vi "Get_Each_channel_reference_samplingdata.vi"(0 "SPU":refnum<k24>, 1 "STSProcess.PDLSTS":refnum<k24>, 2 "Refdata_struct":refnum<k24>[](array[refnum]), 3 "SOP":i32, 5 "Ref_monitordata_struct":refnum<k24>[](array[refnum]), 7 "MPM":refnum<k24>[](array[refnum]), 9 "ChannelNumber":i32, 11 "错误输入（无错误）":errorcluster, 12 "SweepCount":i32, 13 "SlotNumber":i32, 14 "MPMNumber":i32) -> (6 "PDLSTS out":refnum<k24>, 15 "error out":errorcluster)   [LabVIEW 2017]
doc: "Get logging reference data & add in"
uses:
  D:/test/PDLSTS/LV_PDL_Sample/DLL/STSProcess.dll
  DLL/STSProcess.dll
  D:/test/PDLSTS/LV_PDL_Sample/DLL/InstrumentDLL.dll
  DLL/InstrumentDLL.dll
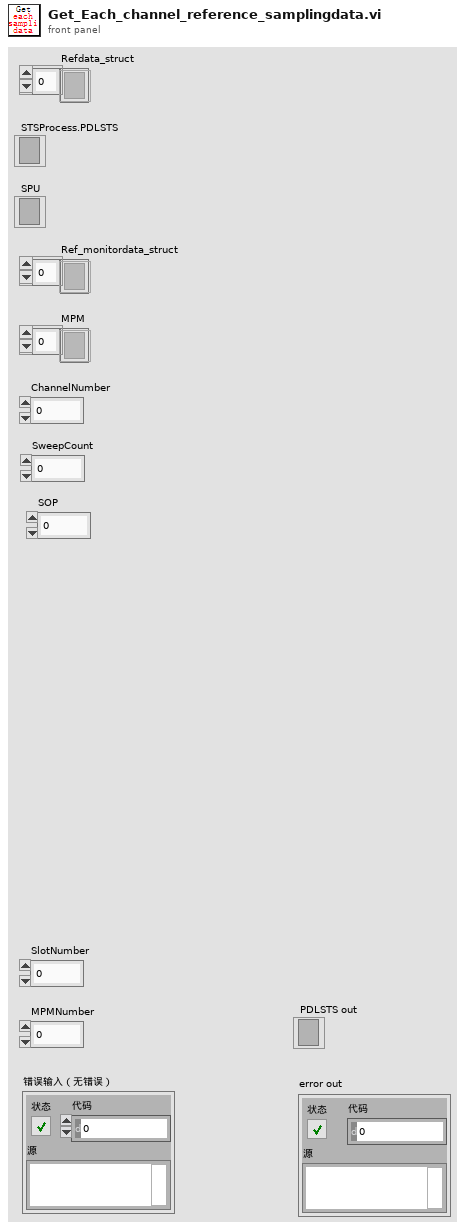
[diagram p1: front panel]
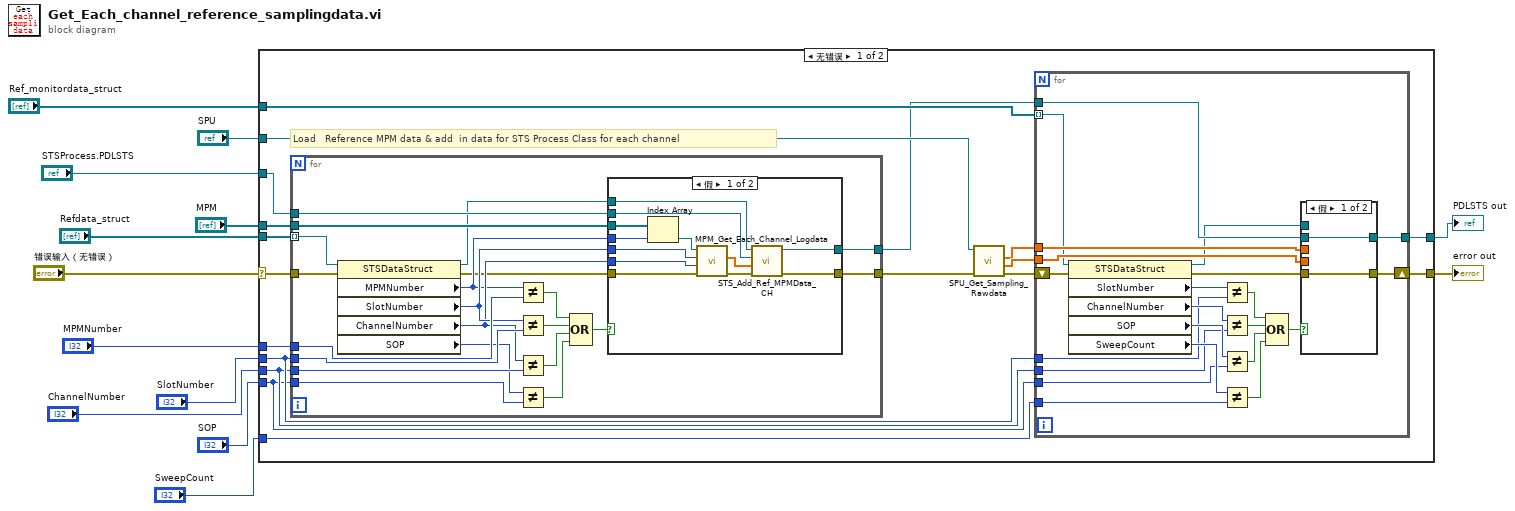
[diagram p0: block diagram]
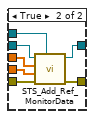
[diagram p2: hidden frame]
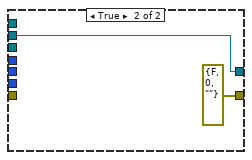
[diagram p3: hidden frame]
diagram:
  n1 = case shown="无错误" "错误输入（无错误）" {
    selector: "错误输入（无错误）" -> [w21 w99]
    tunnel: "STSProcess.PDLSTS" -> [w19 w98]
    tunnel: "Ref_monitordata_struct" -> [w28 _]
    tunnel: "SPU" -> [w27 _]
    tunnel: "MPM" -> [w25 _]
    tunnel: "ChannelNumber" -> [w16 _]
    tunnel: "SlotNumber" -> [w17 _]
    tunnel: "MPMNumber" -> [w24 _]
    tunnel: "Refdata_struct" -> [w23 _]
    tunnel: [w22 w99] -> w5
    tunnel: [w20 w98] -> w3
    tunnel: "SOP" -> [w15 _]
    tunnel: "SweepCount" -> [w14 _]
    frame No Error {
      # "Load　Reference MPM data & add  in data for STS Process Class for each channel"
      n2 = for {
        tunnel: w23 -> [w71] mode=indexing
        tunnel: w24 -> [w83]
        tunnel: w17 -> [w82]
        tunnel: w16 -> [w81]
        tunnel: w25 -> [w74]
        tunnel: w19 -> [w72]
        tunnel: [w70] -> w26
        tunnel: w21 -> [w68]
        tunnel: [w66] -> w18
        tunnel: w15 -> [w64]
        n3 = property on="属性节点" class="STSDataStruct"(reference=w71, error in=w68) -> (reference out=w67:refnum<k24>, error out=w69:errorcluster, "MPMNumber"=w73:i32, "SlotNumber"=w76:i32, "ChannelNumber"=w75:i32, "SOP"=w65:i32)
        n4 = Not Equal?(x=w73, y=w83) -> (x != y?=w80:bool)
        n5 = Not Equal?(x=w76, y=w82) -> (x != y?=w79:bool)
        n6 = Not Equal?(x=w75, y=w81) -> (x != y?=w78:bool)
        n7 = Not Equal?(x=w65, y=w64) -> (x != y?=w63:bool)
        n8 = Compound Arithmetic op=OR ("复合运算")(w80, w79, w78, w63) -> (w77:bool)
        n9 = case shown="假" w77 {
          tunnel: w76 -> [w95 _]
          tunnel: w75 -> [w94 _]
          tunnel: w74 -> [w93 _]
          tunnel: w73 -> [w91 _]
          tunnel: w72 -> [w90 w96]
          tunnel: w67 -> [w89 _]
          tunnel: [w86 errorcluster {"status"=FALSE, "code"=0, "source"=""} ("错误输出")] -> w70
          tunnel: w69 -> [w85 _]
          tunnel: [w84 w96] -> w66
          frame False {
            n10 = Index Array(array=w93, index=w91) -> (element=w92:refnum<k24>)
            n11 = call "MPM_Get_Each_Channel_Logdata.vi"("error in (no error)"=w85, "channelNumber"=w94, "moduleNumber"=w95, ".NET Reference in"=w92) -> ("error out"=w87:errorcluster, "data out"=w88:sgl[])  [unwired: 5 in, 1 out]
            n12 = call "STS_Add_Ref_MPMData_CH.vi"("错误输入（无错误）"=w87, "data"=w88, "STSProcess.PDSTS"=w90, "Setting"=w89) -> ("错误输出"=w86:errorcluster, "PDLSTS"=w84:refnum<k24>)  [unwired: 6 in]
          }
          frame True {
          }
        }
      }
      n13 = call "SPU_Get_Sampling_Rawdata.vi"("错误输入（无错误）"=w26, "SPU"=w27) -> ("error out"=w29:errorcluster, "monitor"=w31:sgl[], "trigger"=w30:sgl[])  [unwired: 5 in, 1 out]
      n14 = for {
        tunnel: w28 -> [w48] mode=indexing
        tunnel: w18 -> [w53]
        tunnel: w30 -> [w52]
        tunnel: w31 -> [w51]
        shift-right: [w50] -> w22
        shift-left: w29 -> [w46]
        tunnel: [w49] -> w20
        tunnel: w17 -> [w35]
        tunnel: w16 -> [w34]
        tunnel: w15 -> [w33]
        tunnel: w14 -> [w32]
        n15 = property class="STSDataStruct"(reference=w48, error in=w46) -> (reference out=w47:refnum<k24>, error out=w45:errorcluster, "SlotNumber"=w39:i32, "ChannelNumber"=w38:i32, "SOP"=w37:i32, "SweepCount"=w36:i32)
        n16 = Not Equal?(x=w39, y=w35) -> (x != y?=w44:bool)
        n17 = Not Equal?(x=w38, y=w34) -> (x != y?=w43:bool)
        n18 = Not Equal?(x=w37, y=w33) -> (x != y?=w42:bool)
        n19 = Not Equal?(x=w36, y=w32) -> (x != y?=w41:bool)
        n20 = Compound Arithmetic op=OR ("复合运算")(w44, w43, w42, w41) -> (w40:bool)
        n21 = case shown="假" w40 {
          tunnel: w53 -> [w55 w62]
          tunnel: w47 -> [_ w61]
          tunnel: w52 -> [_ w60]
          tunnel: w51 -> [_ w59]
          tunnel: w45 -> [w54 w58]
          tunnel: [w54 w57] -> w50
          tunnel: [w55 w56] -> w49
          frame False {
          }
          frame True {
            n22 = call "STS_Add_Ref_MonitorData.vi"("setting"=w61, "错误输入（无错误）"=w58, "monitorData"=w59, "triggerIndex"=w60, "STSProcess.PDLSTS"=w62) -> ("错误输出"=w57:errorcluster, "PDLSTS out"=w56:refnum<k24>)  [unwired: 5 in]
          }
        }
      }
    }
    frame Error {
    }
  }
  "error out" <- w5
  "PDLSTS out" <- w3
